vi "AVI play.vi"(0 "RGB Image ref":T5, 1 "Number of Frames":u32, 2 "Stop button pressed":bool, 4 "I16 Image ref":T5, 5 "error in (no error)":errorcluster, 6 "AVI modes refs in":T2, 7 "AVI mode":T1, 8 "Frame number (in)":i32) -> (13 "Playback stopped":bool, 14 "I16 image ref out":T5, 16 "Speed data waveform graph":dbl[](graph), 17 "Frame number (out)":i32, 18 "AVI modes refs out":T2, 19 "error out":errorcluster)   [LabVIEW 2020]
uses:
  <vilib>/vision/Image Controls.llb/IMAQ Image.ctl
  Typedefs/AVI modes refs cluster.ctl
  <vilib>/vision/Avi1.llb/AviRefnum.ctl
  <vilib>/vision/Avi.llb/IMAQ AVI2 Refnum.ctl
  Typedefs/AVI implementation enum.ctl
  Typedefs/Select Play-Stop button to show.ctl
  Globals/gl_Time series viewer globals.vi
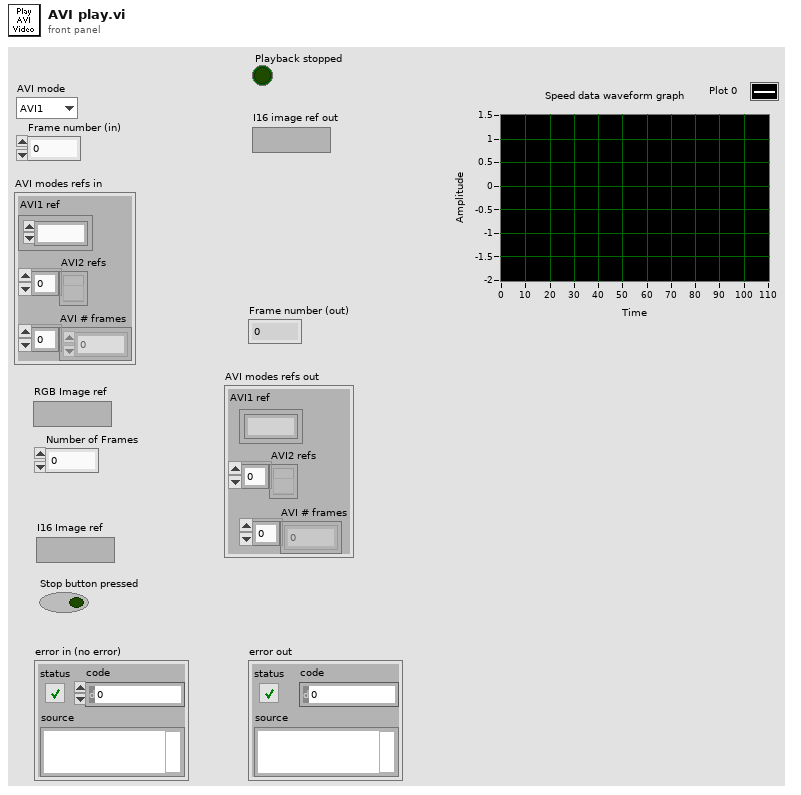
[diagram p1: front panel]
types:
  T1 = typedef "AVI implementation enum.ctl" = enum16{"AVI1", "AVI2"}
  T2 = typedef "AVI modes refs cluster.ctl" = cluster{"AVI1 ref":T3, "AVI2 refs":T4[], "AVI # frames":u32[]}
  T3 = typedef "AviRefnum.ctl" = refnum<k1>
  T4 = typedef "IMAQ AVI2 Refnum.ctl" = refnum<k20>
  T5 = typedef "IMAQ Image.ctl" = refnum<image>
  T6 = typedef "Time series viewer refs.ctl" = cluster{"This VI":refnum<vi>, "Image control":refnum<vi>, "AVI Mode ind":refnum<vi>, "Play":refnum<vi>, "Stop":refnum<vi>, "Back":refnum<vi>, "Scrollbar":refnum<vi>, "Video length info":refnum<vi>, "Expected speed values":refnum<vi>, "Intensity":refnum<vi>, "Path":refnum<vi>, "Selection sliders":refnum<vi>, "Speed Graph ref":refnum<vi>, "Frame rate set (fps)":refnum<vi>, "Number of rows to generate":refnum<vi>, "VL Image Array":refnum<vi>, "Image Scrollbar":refnum<vi>, "Channel to load":refnum<vi>, "Colour":refnum<vi>}
  T7 = typedef "Select Play-Stop button to show.ctl" = enum16{"Show Play button", "Show Stop button"}
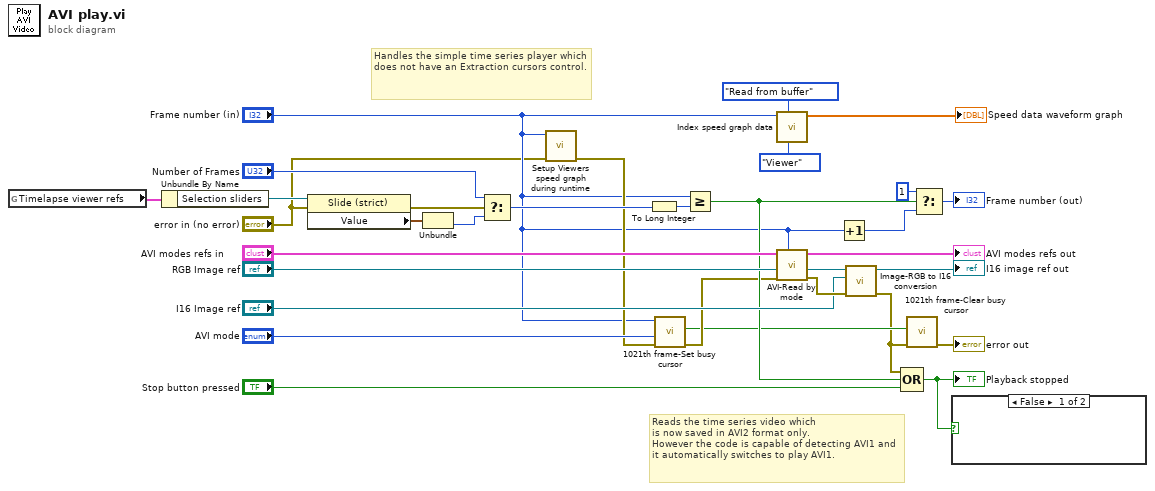
[diagram p0: block diagram]
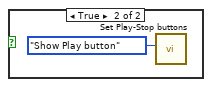
[diagram p2: hidden frame]
diagram:
  # "Handles the simple time series player which does not have an Extraction cursors control."
  # "Reads the time series video which \nis now saved in AVI2 format only.\nHowever the code is capable of detecting AVI1 and it automatically switches to play AVI1."
  n1 = global read "gl_Time series viewer globals.vi" "Timelapse viewer refs"() -> (w5:T6)
  n2 = Unbundle By Name(w5) -> ("Selection sliders"=w13:refnum<vi>)
  n3 = property class="Slide (strict)"(reference=w13, error in="error in (no error)") -> (error out=w4:errorcluster, "Value"=w12:cluster{i32, i32})  [unwired: 1 out]
  n4 = Unbundle(w12) -> (w11:i32)  [unwired: 1 out]
  n5 = Select(t="Number of Frames", s=w4, f=w11) -> (s? t:f=w10:u32)
  n6 = call "Setup Viewers speed graph during runtime.vi"("error in (no error)"="error in (no error)", "Frame number or cycle number"="Frame number (in)") -> ("error out"=w3:errorcluster)  [unwired: 9 in]
  n7 = To Long Integer(number=w10) -> (32bit integer=w19:i32)
  n8 = call "1021th frame-Set busy cursor.vi"("error in (no error)"=w3, "AVI mode"="AVI mode", "Frame number"="Frame number (in)") -> ("error out"=w17:errorcluster, "Busy cursor was set"=w16:bool)  [unwired: 7 in]
  n9 = Greater Or Equal?(x="Frame number (in)", y=w19) -> (x >= y?=w24:bool)
  n10 = call "Index speed graph data.vi"("Caller"=enum16{"Viewer", "Exporter"}."Viewer", "Buffer operation (read from internal buffer)"=enum16{"Update buffer", "Read from buffer"}."Read from buffer", "Gobal frame number in Timelapse data/master video (1 based)"="Frame number (in)") -> ("Speed data waveform graph"=→"Speed data waveform graph":dbl[])  [unwired: 6 in, 2 out]
  n11 = call "AVI-Read by mode.vi"("Frame number (unity-based)"="Frame number (in)", "error in (no error)"=w17, "RGB image ref in"="RGB Image ref", "AVI modes refs"="AVI modes refs in") -> ("error out"=w31:errorcluster, "RGB image ref out"=w28:T5, "AVI modes refs"=→"AVI modes refs out":T2)  [unwired: 5 in]
  n12 = Increment(x="Frame number (in)") -> (x+1=w32:i32)
  n13 = call "Image-RGB to I16 conversion.vi"("error in (no error)"=w31, "I16 image ref in"="I16 Image ref", "RGB image ref in"=w28) -> ("error out"=w15:errorcluster, "I16 image ref out"=→"I16 image ref out":T5)  [unwired: 7 in]
  n14 = Compound Arithmetic op=OR(w15, w24, "Stop button pressed") -> (w20:bool)
  "Playback stopped" <- w20
  n15 = call "1021th frame-Clear busy cursor.vi"("error in (no error)"=w15, "Busy cursor was set"=w16) -> ("error out"=→"error out":errorcluster)  [unwired: 9 in]
  n16 = Select(t=1, s=w24, f=w32) -> (s? t:f=→"Frame number (out)":i32)
  n17 = case shown="False" w20 {
    frame False {
    }
    frame True {
      n18 = call "Set Play-Stop buttons.vi"("Function"=Select_Play-Stop_button_to_show."Show Play button") -> ()  [unwired: 10 in, 1 out]
    }
  }
